vi "VISA Test.vi"() -> ()   [LabVIEW 2018]
panel:
  in  "Open":bool
  in  "Get ID":bool
  out "ID":string
  in  "error in (no error)":errorcluster
  out "error out":errorcluster
  in  "VISA resource":refnum<visa-resource-name>
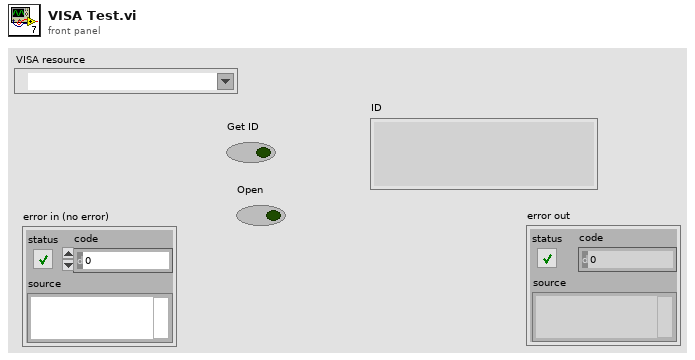
[diagram p1: front panel]
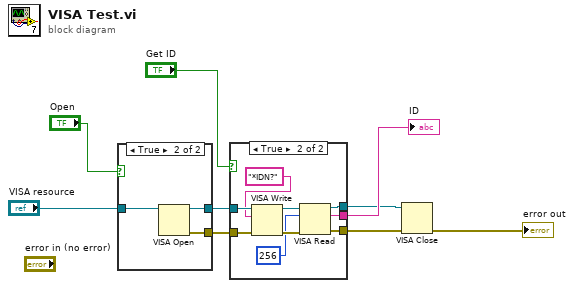
[diagram p0: block diagram]
diagram:
  n1 = case shown="True" "Open" {
    tunnel: "VISA resource" -> [w10 w13]
    tunnel: [w10 w12] -> w8
    tunnel: [_ w11] -> w7
    frame False {
    }
    frame True {
      n2 = VISA Open(VISA resource name=w13) -> (VISA resource name=w12:refnum<visa-resource-name>, error out=w11:errorcluster)  [unwired: 4 in]
    }
  }
  n3 = case shown="True" "Get ID" {
    tunnel: w8 -> [w15 w23]
    tunnel: w7 -> [w14 w24]
    tunnel: [_ w20] -> w6
    tunnel: [w15 w19] -> w5
    tunnel: [w14 w18] -> w4
    frame False {
    }
    frame True {
      n4 = VISA Write(VISA resource name=w23, write buffer="*IDN?", error in (no error)=w24) -> (VISA resource name out=w21:refnum<visa-resource-name>, error out=w22:errorcluster)  [unwired: 1 out]
      n5 = VISA Read(VISA resource name=w21, byte count=u32 256, error in (no error)=w22) -> (VISA resource name out=w19:refnum<visa-resource-name>, read buffer=w20:string, error out=w18:errorcluster)  [unwired: 1 out]
    }
  }
  "ID" <- w6
  n6 = VISA Close(VISA resource name=w5, error in (no error)=w4) -> (error out=→"error out":errorcluster)
